vi "Oculus Rift Controller().vi"() -> (3 "Controller Library:Oculus Rift Controller.lvclass":refnum<class "Oculus Rift Controller.lvclass">)   [LabVIEW 2014, in "Controller Library.lvlib" / "Oculus Rift Controller.lvclass"]
uses:
  Oculus Rift Controller.lvclass
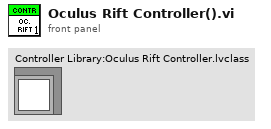
[diagram p1: front panel]
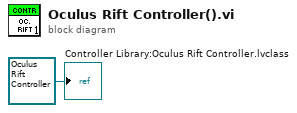
[diagram p0: block diagram]
diagram:
  "Controller Library:Oculus Rift Controller.lvclass" <- refnum<class "Oculus Rift Controller.lvclass"> refnum ("Controller Library:Oculus Rift Controller.lvclass")
